vi "Detect Change.vi"(8 "Error In":errorcluster, 10 "Frame":u32[][](array[colorbox]), 11 "Display In":refnum<class "Neopixel - Host.lvclass">) -> (0 "Error Out":errorcluster, 2 "Frame Change":bool, 3 "Display Out":refnum<class "Neopixel - Host.lvclass">)   [LabVIEW 2021, in "Neopixel - Host.lvclass"]
uses:
  Neopixel - Host.lvclass
  Neopixel - Host.lvclass/Neopixel - Host.ctl
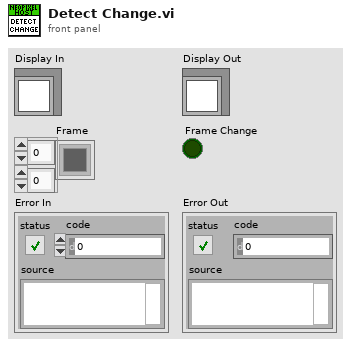
[diagram p1: front panel]
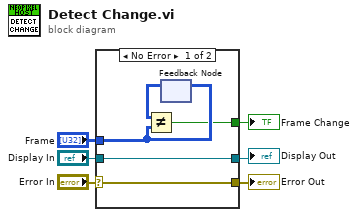
[diagram p0: block diagram]
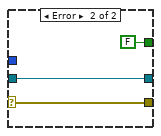
[diagram p2: hidden frame]
diagram:
  n1 = case shown="No Error" "Error In" {
    selector: "Error In" -> [w7 w13]
    tunnel: "Display In" -> [w8 w14]
    tunnel: [w7 w13] -> w4
    tunnel: [w8 w14] -> w3
    tunnel: "Frame" -> [w10 _]
    tunnel: [w9 FALSE] -> w1
    frame No Error {
      n2 = feedback #1() -> (w11:u32[][])  [unwired: 1 in]
      n3 = Not Equal?(x=w11, y=w10) -> (x != y?=w9:bool)
      n4 = feedback-in #1(w10) -> ()
    }
    frame Error {
    }
  }
  "Error Out" <- w4
  "Display Out" <- w3
  "Frame Change" <- w1
